vi "Build Error Cluster__ogtk.vi"(1 "String to Prepend to source (\"\")":string, 2 "code":i32) -> (0 "error out":errorcluster)   [LabVIEW 2016]
doc: "Creates an error cluster, building the source string from the calling VIs call chain in a standard LabVIEW fashon. Builds source string as:\n\n\"<B>Calling VI</B> in <B>Calling VI's Caller</B>-><B>Calling VI's Caller's Caller</B>->etc...->etc...\"\n\nOptional 'String to Prepend to source (\"\")' string input is used to add extra descriptive info to the source string. This string, if present, will be enclosed in parenthesis and prepended to the source string."
panel:
  # "[OpenG VI Tags] ***Do Not Remove***"
  # "Build Error Cluster.vi\n\nCreates an error cluster, building the source string from the calling VIs call chain in a standard LabVIEW fashon.\n\nPlease visit http://www.OpenG.org to learn about the\nOpen Source LabVIEW software movement.\n\nNOTICE -- YOU MUST LEAVE THIS NOTICE IN PLACE.  PER THE TERMS OF THE LICENSE BELOW, YOU MAY SUBLICENSE THIS SOFTWARE \nIN ANY WAY THAT DOES NOT CONFLICT WITH THIS LICENSE.\n\n### BSD License (http://www.opensource.org/licenses/bsd-license.php) Begin ###\n \nCopyright (c) 2002-2006, Jim Kring <jim@jimkring.com>\n\nAll rights reserved.\n\nRedistribution and use in source and binary forms, with or without modification, are permitted provided that the following conditions are met:\n\n    * Redistributions of source code must retain the above copyright notice, this list of conditions and the following disclaimer.\n    * Redistributions in binary form must reproduce the above copyright notice, this list of conditions and the following disclaimer in the \n       documentation and/or other materials provided with the distribution.\n    * Neither the name of SciWare, James Kring, Inc., nor the names of its contributors may be used to endorse or promote products derived \n       from this software without specific prior written permission.\n\nTHIS SOFTWARE IS PROVIDED BY THE COPYRIGHT HOLDERS AND CONTRIBUTORS \"AS IS\" AND ANY EXPRESS OR IMPLIED WARRANTIES, \nINCLUDING, BUT NOT LIMITED TO, THE IMPLIED WARRANTIES OF MERCHANTABILITY AND FITNESS FOR A PARTICULAR PURPOSE ARE \nDISCLAIMED. IN NO EVENT SHALL THE COPYRIGHT OWNER OR CONTRIBUTORS BE LIABLE FOR ANY DIRECT, INDIRECT, INCIDENTAL,\n SPECIAL, EXEMPLARY, OR CONSEQUENTIAL DAMAGES (INCLUDING, BUT NOT LIMITED TO, PROCUREMENT OF SUBSTITUTE GOODS OR \nSERVICES; LOSS OF USE, DATA, OR PROFITS; OR BUSINESS INTERRUPTION) HOWEVER CAUSED AND ON ANY THEORY OF LIABILITY, \nWHETHER IN CONTRACT, STRICT LIABILITY, OR TORT (INCLUDING NEGLIGENCE OR OTHERWISE) ARISING IN ANY WAY OUT OF THE USE \nOF THIS SOFTWARE, EVEN IF ADVISED OF THE POSSIBILITY OF SUCH DAMAGE.\n\n### BSD License End ###"
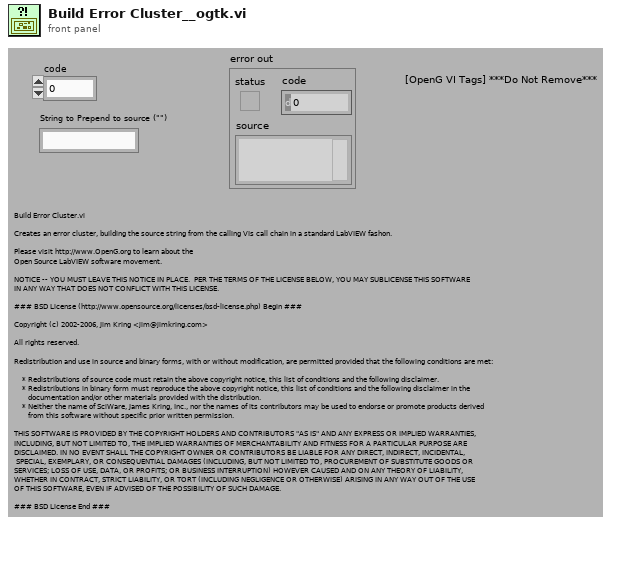
[diagram p1: front panel]
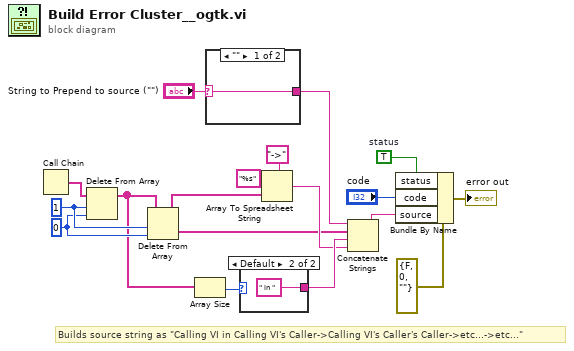
[diagram p0: block diagram]
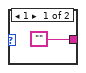
[diagram p2: hidden frame]
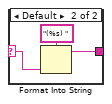
[diagram p3: hidden frame]
diagram:
  w12 = 0 ("Index")
  w13 = 1 ("Length")
  w8 = TRUE  # status
  # "Builds source string as \"Calling VI in Calling VI's Caller->Calling VI's Caller's Caller->etc...->etc...\""
  n1 = Call Chain() -> (call chain=w18:string[])
  n2 = Delete From Array(array=w18, length=w13, index=w12) -> (array with subset deleted=w1:string[])  [unwired: 1 out]
  n3 = Delete From Array(array=w1, length=w13, index=w12) -> (deleted portion=w2:string[], array with subset deleted=w11:string[])
  n4 = Array Size(array=w1) -> (size(s)=w3:i32)
  n5 = case shown="\"\"" "String to Prepend to source (\"\")" {
    selector: "String to Prepend to source (\"\")" -> [w19 w22]
    tunnel: [w19 w20] -> w4
    frame "" {
    }
    frame Default {
      n6 = Format Into String(format string="(%s) " ("Format String"), w22) -> (resulting string=w20:string)  [unwired: 2 in, 1 out]
    }
  }
  n7 = case shown="Default" w3 {
    tunnel: ["" " in " ("Format String")] -> w16
    frame 1 {
    }
    frame Default {
    }
  }
  n8 = Array To Spreadsheet String(delimiter (Tab)="->", array=w11, 3:"%s" ("format string")) -> (spreadsheet string=w15:string)
  n9 = Concatenate Strings(w4, w2, w16, w15) -> (w7:string)
  n10 = Bundle By Name(cluster=errorcluster {"status"=FALSE, "code"=0, "source"=""} ("error out"), "status"=w8, "code"="code", "source"=w7) -> (→"error out":errorcluster)
